vi "Tabulate_FFID_Bkgnd_Volts.vi"() -> ()   [LabVIEW 2014]
uses:
  Controls/File_Selector_Type.ctl
  Controls/Post_Process.ctl
  Controls/Setup.ctl
  Controls/Save_Data.ctl
  Globals/Meas_global.vi
panel:
  in  "At Dialog Prompt Post Process":T1=enum."Files containing the search string in the selected folder"
  in  "Search String":string="FF_Bkgnd_"
  out "current index":i32
  out "No Of files":i32
  in  "Raw Data folder":path
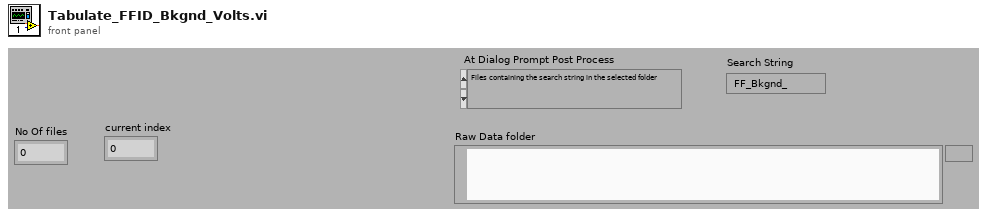
[diagram p1: front panel]
types:
  T1 = typedef "File_Selector_Type.ctl" = enum16{"The Selected File", "The Selected Folder", "Files containing the search string in the selected folder", "All files listed in selected file"}
  T2 = typedef "Save_Data.ctl" = enum16{"Save No Data", "Save Data"}
  T3 = typedef "Setup.ctl" = enum16{"Run Program", "Show Setup", "Save Current Setup", "Setup Front Panel"}
  T4 = typedef "Post_Process.ctl" = enum16{"Take New Data", "Post Process Raw Data File"}
  T5 = typedef "Analysis_info_cluster.ctl" = cluster{"Colour":u32, "Inst type":T6, "Inst name":string, "Symbol":string, "Code name":string, "Extra Info":string, "Inst Array":T7, "Extra Titles":string[], "Extra Values":string[], "U":dbl, "u^2":dbl, "u^3":dbl, "u^4":dbl, "Skew_u":dbl, "Kurt_u":dbl, "Sd Error in Mean":dbl, "% u'/U":dbl, "X":dbl, "Y":dbl, "Z":dbl, "Timescale integral to 25%":dbl, "Sd Error in Variance":dbl, "Calib File":path, "Calib Constants":dbl[], "Output Position":bool, "Full Stats":bool, "Av Sampling Rate":dbl, "Av No of Samples":dbl, "Total Meas Time (s)":dbl, "ADAM Ch Name":string}
  T6 = typedef "Inst_type.ctl" = enum16{"Propeller anemometer", "Raw voltage", "Pressure Transducer", "Pitot-static tube", "Preston tube", "Hot wire", "Cross wire 1", "Cross wire 2", "Generic Linear", "Generic Polynomial", "Generic BackPoly", "Fast FID", "Thermocouple", "Cold wire", "Pulsed Wire", "LDA Vel", "LDA Tran time", "LDA Arr time"}
  T7 = typedef "Instrument_Array.ctl" = enum16{"PWA", "LDA", "Analogue"}
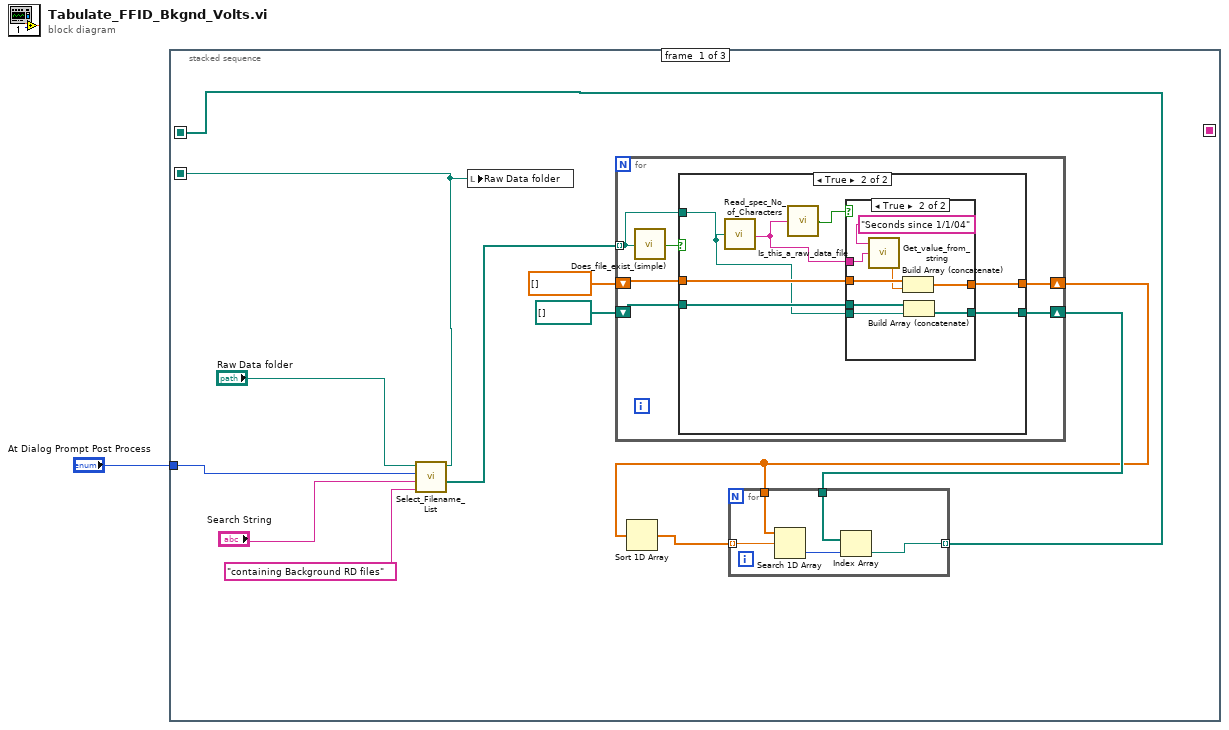
[diagram p0: block diagram]
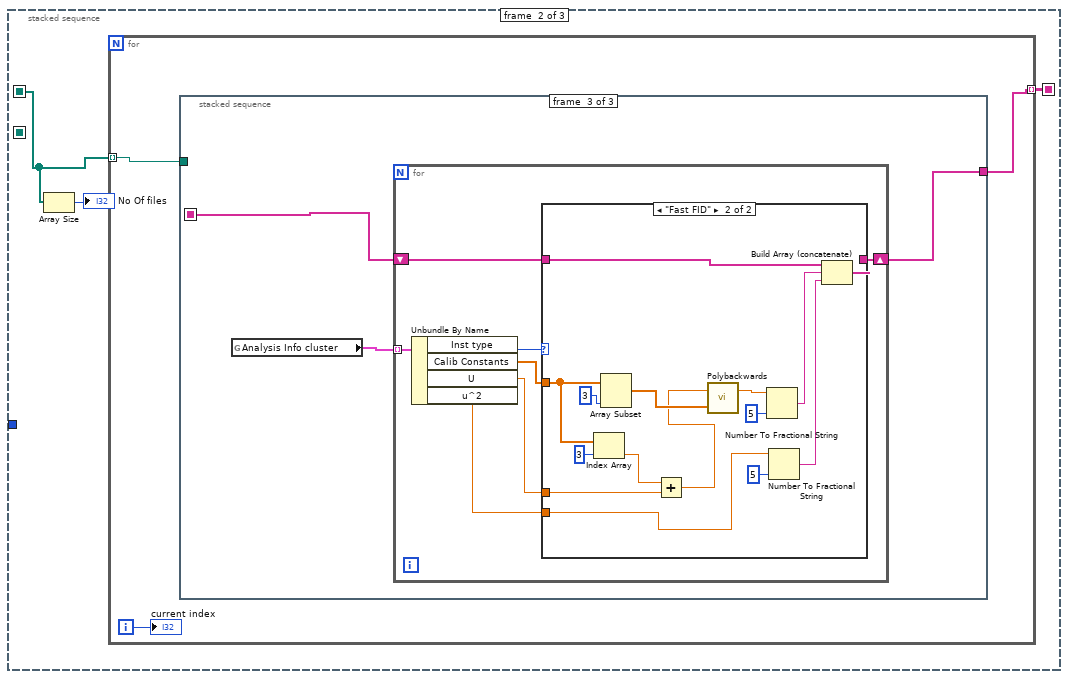
[diagram p4: hidden frame]
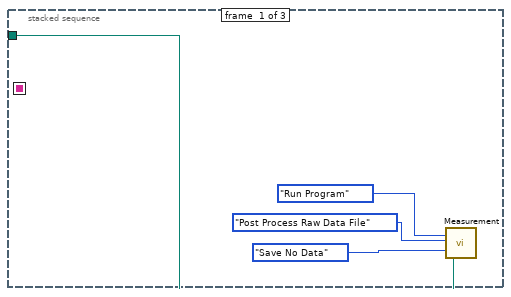
[diagram p5: hidden frame]
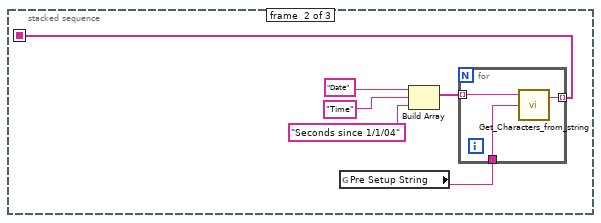
[diagram p6: hidden frame]
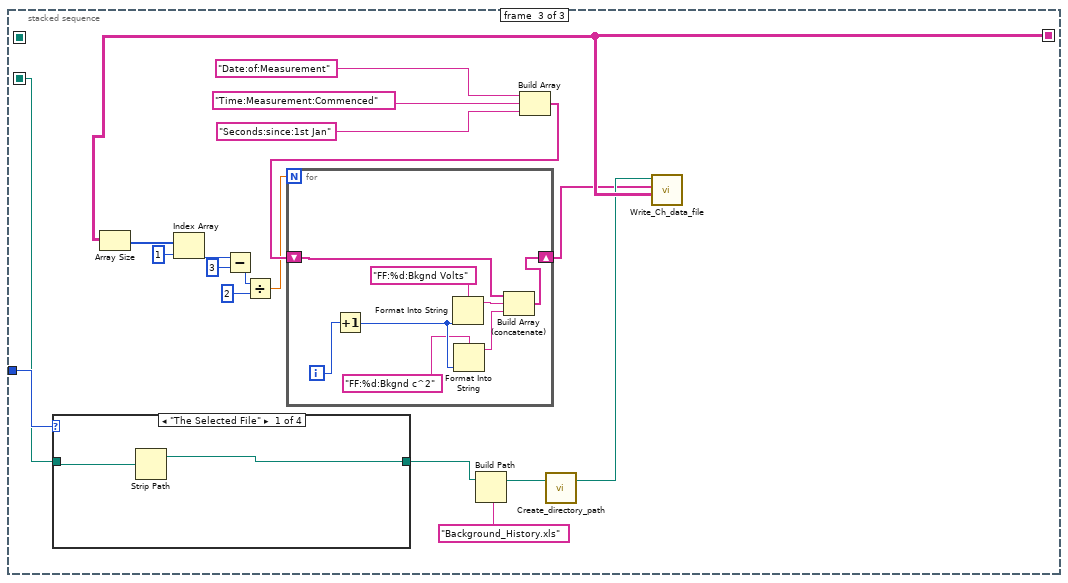
[diagram p8: hidden frame]
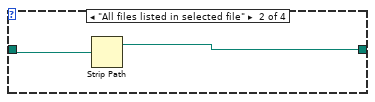
[diagram p9: hidden frame]
diagram:
  n1 = stacked-sequence {
    seq-local: [_ w44 _] -> [_ _ w100]
    seq-local: [w10 _ _] -> [_ _ w94]
    seq-local: [w3 _ _] -> [_ w45 _]
    tunnel: "At Dialog Prompt Post Process" -> [w2 _ w96]
    frame #0 {
      n2 = call "Select_Filename_List.vi"("File Type"="containing Background RD files", "Search String"="Search String", "At Dialog Prompt Post Process"=w2, "Previous Choice"="Raw Data folder") -> ("Selected files"=w4:path[], "Choosen path"=w10:path)  [unwired: 1 in, 2 out]
      n3 = local write "Raw Data folder"(w10) -> ()
      n4 = for {
        tunnel: w4 -> [w19] mode=indexing
        shift-right: [w23] -> w5
        shift-left: dbl[] [] -> [w24]
        shift-right: [w21] -> w8
        shift-left: path[] [] -> [w22]
        n5 = call "Does_file_exist_(simple).vi"("Pathname"=w19) -> ("exists?"=w20:bool)
        n6 = case shown="True" w20 {
          tunnel: w24 -> [w26 w33]
          tunnel: [w26 w32] -> w23
          tunnel: w22 -> [w25 w31]
          tunnel: [w25 w30] -> w21
          tunnel: w19 -> [_ w28]
          frame False {
          }
          frame True {
            n7 = call "Read_spec_No_of_Characters.vi"("Filename"=w28) -> ("character string"=w27:string)  [unwired: 1 out]
            n8 = call "Is_this_a_raw_data_file.vi"("character string"=w27) -> ("Raw Dat File?"=w29:bool)  [unwired: 2 out]
            n9 = case shown="True" w29 {
              tunnel: w33 -> [w35 w41]
              tunnel: [w35 w43] -> w32
              tunnel: w31 -> [w34 w39]
              tunnel: w28 -> [_ w38]
              tunnel: [w34 w37] -> w30
              tunnel: w27 -> [_ w36]
              frame False {
              }
              frame True {
                n10 = call "Get_value_from_string.vi"("Input string"=w36, "Variable name"="Seconds since 1/1/04") -> ("Value"=w40:dbl)  [unwired: 1 in, 1 out]
                n11 = Build Array (concatenate)(w41, w40) -> (w43:dbl[])
                n12 = Build Array (concatenate)(w39, w38) -> (w37:path[])
              }
            }
          }
        }
      }
      n13 = Sort 1D Array(array=w5) -> (sorted array=w6:dbl[])
      n14 = for {
        tunnel: w5 -> [w18]
        tunnel: w6 -> [w17] mode=indexing
        tunnel: w8 -> [w16]
        tunnel: [w15] -> w3 mode=indexing
        n15 = Search 1D Array(1D array=w18, element=w17) -> (index of element=w14:i32)  [unwired: 1 out]
        n16 = Index Array(array=w16, index=w14) -> (element=w15:path)
      }
    }
    frame #1 {
      n17 = Array Size(array=w45) -> (size(s)=→"No Of files":i32)
      n18 = for {
        tunnel: w45 -> [w49] mode=indexing
        tunnel: [w47] -> w44 mode=indexing
        i -> [w48]
        n19 = stacked-sequence {
          seq-local: [_ w54 _] -> [_ _ w64]
          tunnel: w49 -> [w50 _ _]
          tunnel: [_ _ w63] -> w47
          frame #0 {
            n20 = call "Measurement.vi"("setup"=Setup."Run Program", "Post Process"=Post_Process."Post Process Raw Data File", "File"=Save_Data."Save No Data", "Raw data file"=w50) -> ()  [unwired: 3 in, 13 out]
          }
          frame #1 {
            n21 = global read "Meas_global.vi" "Pre Setup String"() -> (w55:string)
            n22 = Build Array("Date", "Time", "Seconds since 1/1/04") -> (w56:string[])
            n23 = for {
              tunnel: w56 -> [w62] mode=indexing
              tunnel: w55 -> [w61]
              tunnel: [w60] -> w54 mode=indexing
              n24 = call "Get_Characters_from_string.vi"("Input string"=w61, "Variable name"=w62) -> ("Value"=w60:string)  [unwired: 1 in, 1 out]
            }
          }
          frame #2 {
            n25 = global read "Meas_global.vi" "Analysis Info cluster"() -> (w65:T5[])
            n26 = for {
              tunnel: w65 -> [w69] mode=indexing
              shift-right: [w70] -> w63
              shift-left: w64 -> [w71]
              n27 = Unbundle By Name(w69) -> ("Inst type"=w72:T6, "Calib Constants"=w68:dbl[], "U"=w67:dbl, "u^2"=w66:dbl)
              n28 = case shown="\"Fast FID\"" w72 {
                tunnel: w68 -> [_ w84]
                tunnel: w71 -> [w73 w81]
                tunnel: [w73 w78] -> w70
                tunnel: w67 -> [_ w75]
                tunnel: w66 -> [_ w74]
                frame "Propeller anemometer", Default {
                }
                frame "Fast FID" {
                  n29 = Index Array(array=w84, index=3 ("Index")) -> (element=w85:dbl)
                  n30 = Array Subset(array=w84, length=3 ("index")) -> (w88:dbl[])  [unwired: 1 in]
                  n31 = Add(x=w85, y=w75) -> (x+y=w83:dbl)
                  n32 = call "Polybackwards.vi"("Coefficients"=w88, "Y input"=w83) -> ("X output"=w79:dbl)  [unwired: 1 out]
                  n33 = Number To Fractional String(number=w79, precision (6)=i16 5) -> (F-format string=w80:string)  [unwired: 2 out]
                  n34 = Number To Fractional String(number=w74, precision (6)=i16 5) -> (F-format string=w76:string)  [unwired: 2 out]
                  n35 = Build Array (concatenate)(w81, w80, w76) -> (w78:string[])
                }
              }
            }
          }
        }
        "current index" <- w48
      }
    }
    frame #2 {
      n36 = case shown="\"The Selected File\"" w96 {
        tunnel: [w108 w110 w112 w113] -> w95
        tunnel: w94 -> [w109 w111 w112 w113]
        frame "The Selected File" {
          n37 = Strip Path(path=w109) -> (stripped path=w108:path)  [unwired: 1 out]
        }
        frame "All files listed in selected file" {
          n38 = Strip Path(path=w111) -> (stripped path=w110:path)  [unwired: 1 out]
        }
        frame "Files containing the search string in the selected folder" {
        }
        frame "The Selected Folder" {
        }
      }
      n39 = Array Size(array=w100) -> (size(s)=w107:i32[])
      n40 = Index Array(array=w107, index=1) -> (element=w101:i32)
      n41 = Subtract(x=w101, y=3) -> (x-y=w91:i32)
      n42 = Divide(x=w91, y=2) -> (x/y=w90:dbl)
      n43 = Build Path(base path=w95, name or relative path="Background_History.xls") -> (appended path=w98:path)
      n44 = Build Array("Date:of:Measurement", "Time:Measurement:Commenced", "Seconds:since:1st Jan") -> (w93:string[])
      n45 = for {
        N: w90 -> [_]
        shift-right: [w115] -> w92
        shift-left: w93 -> [w116]
        i -> [w121]
        n46 = Increment(x=w121) -> (x+1=w119:i32)
        n47 = Format Into String(format string="FF:%d:Bkgnd Volts", w119) -> (resulting string=w118:string)  [unwired: 2 in, 1 out]
        n48 = Format Into String(format string="FF:%d:Bkgnd c^2", w119) -> (resulting string=w117:string)  [unwired: 2 in, 1 out]
        n49 = Build Array (concatenate)(w116, w118, w117) -> (w115:string[])
      }
      n50 = call "Create_directory_path.vi"("Path name"=w98) -> ("Path name Out"=w97:path)  [unwired: 1 in, 1 out]
      n51 = call "Write_Ch_data_file.vi"("Channel Values"=w100, "Channel names"=w92, "Filename"=w97) -> ()  [unwired: 5 in, 4 out]
    }
  }
